vi "MotorTestBench_Main.vi"() -> ()   [LabVIEW 2026]
uses:
  MotorMeasurements.ctl
  FaultInjectionMode.ctl
  <vilib>/Plasmionique/MB Master/MB_Master_TCP/MB_Master_TCP.lvclass
  C:/Program Files/National Instruments/LabVIEW 2026/vi.lib/Plasmionique/MB Master/MB_Master/MB_Master.lvclass
panel:
  in  "Fault Injection":T1
  out "Modbus System Status":u16
  in  "Timeout":i32=10000
  in  "Slave ID":u8=255
  in  "Port":u16=502
  in  "IP Address":string="localhost"
  in  "Test Vibration \nLimit (mm/s)":dbl
  in  "Safety Vibration\nTrip (mm/s)":dbl
  out "Vibration OK":bool
  in  "Measurement\nSource":T2(ring)
  out "Measurements":T3
  in  "ai0 = Temperature\nai1 = Current\nai2 = Torque\nai3 = Vibration\nai4 = RPM":tag
  out "RPM Error":dbl
  out "Test Result":string
  in  "RESET TEST":bool
  in  "Safety Current\nTrip (A)":dbl
  in  "Safety Temp.\nTrip (°C)":dbl
  out "TEST FAILED":bool
  out "Current OK":bool
  out "RPM OK":bool
  in  "Test Current\nLimit (A)":dbl
  in  "RPM Tolerance":dbl
  out "Temprature OK":bool
  in  "Test Temperature\nLimit (°C)":dbl
  in  "START TEST":bool
  out "Current Test State":T4(ring)
  in  "STOP SYSTEM":bool
  # "SETTINGS"
  # "MOTOR TEST BENCH"
  # "DAQ Channel Selection"
  # "TEST CONTROL"
  # "LIVE MEASUREMENTS"
  # "LIMITS"
  # "MODBUS SETTINGS"
  # "FAULT / STATUS"
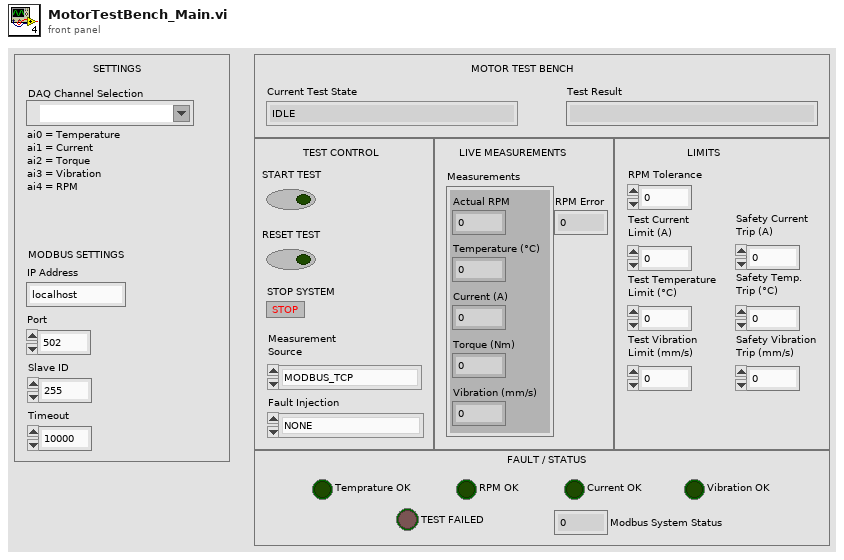
[diagram p1: front panel]
types:
  T1 = typedef "FaultInjectionMode.ctl" = enum16{"NONE", "OVERCURRENT", "OVERTEMPERATURE", "HIGH_VIBRATION", "RPM_SENSOR_FAILURE"}
  T2 = enum16{"MODBUS_TCP", "NI_DAQ", "SOFTWARE_SIMULATOR"}
  T3 = typedef "MotorMeasurements.ctl" = cluster{"Temperature (°C)":dbl, "Current (A)":dbl, "Torque (Nm)":dbl, "Vibration (mm/s)":dbl, "Actual RPM":dbl}
  T4 = enum16{"IDLE", "TEST_1000_RPM", "TEST_2000_RPM", "TEST_3000_RPM", "COMPLETE", "FAULT", "SHUTDOWN"}
  T5 = enum16{"open", "open or create", "create or replace", "create", "open (read-only)"}
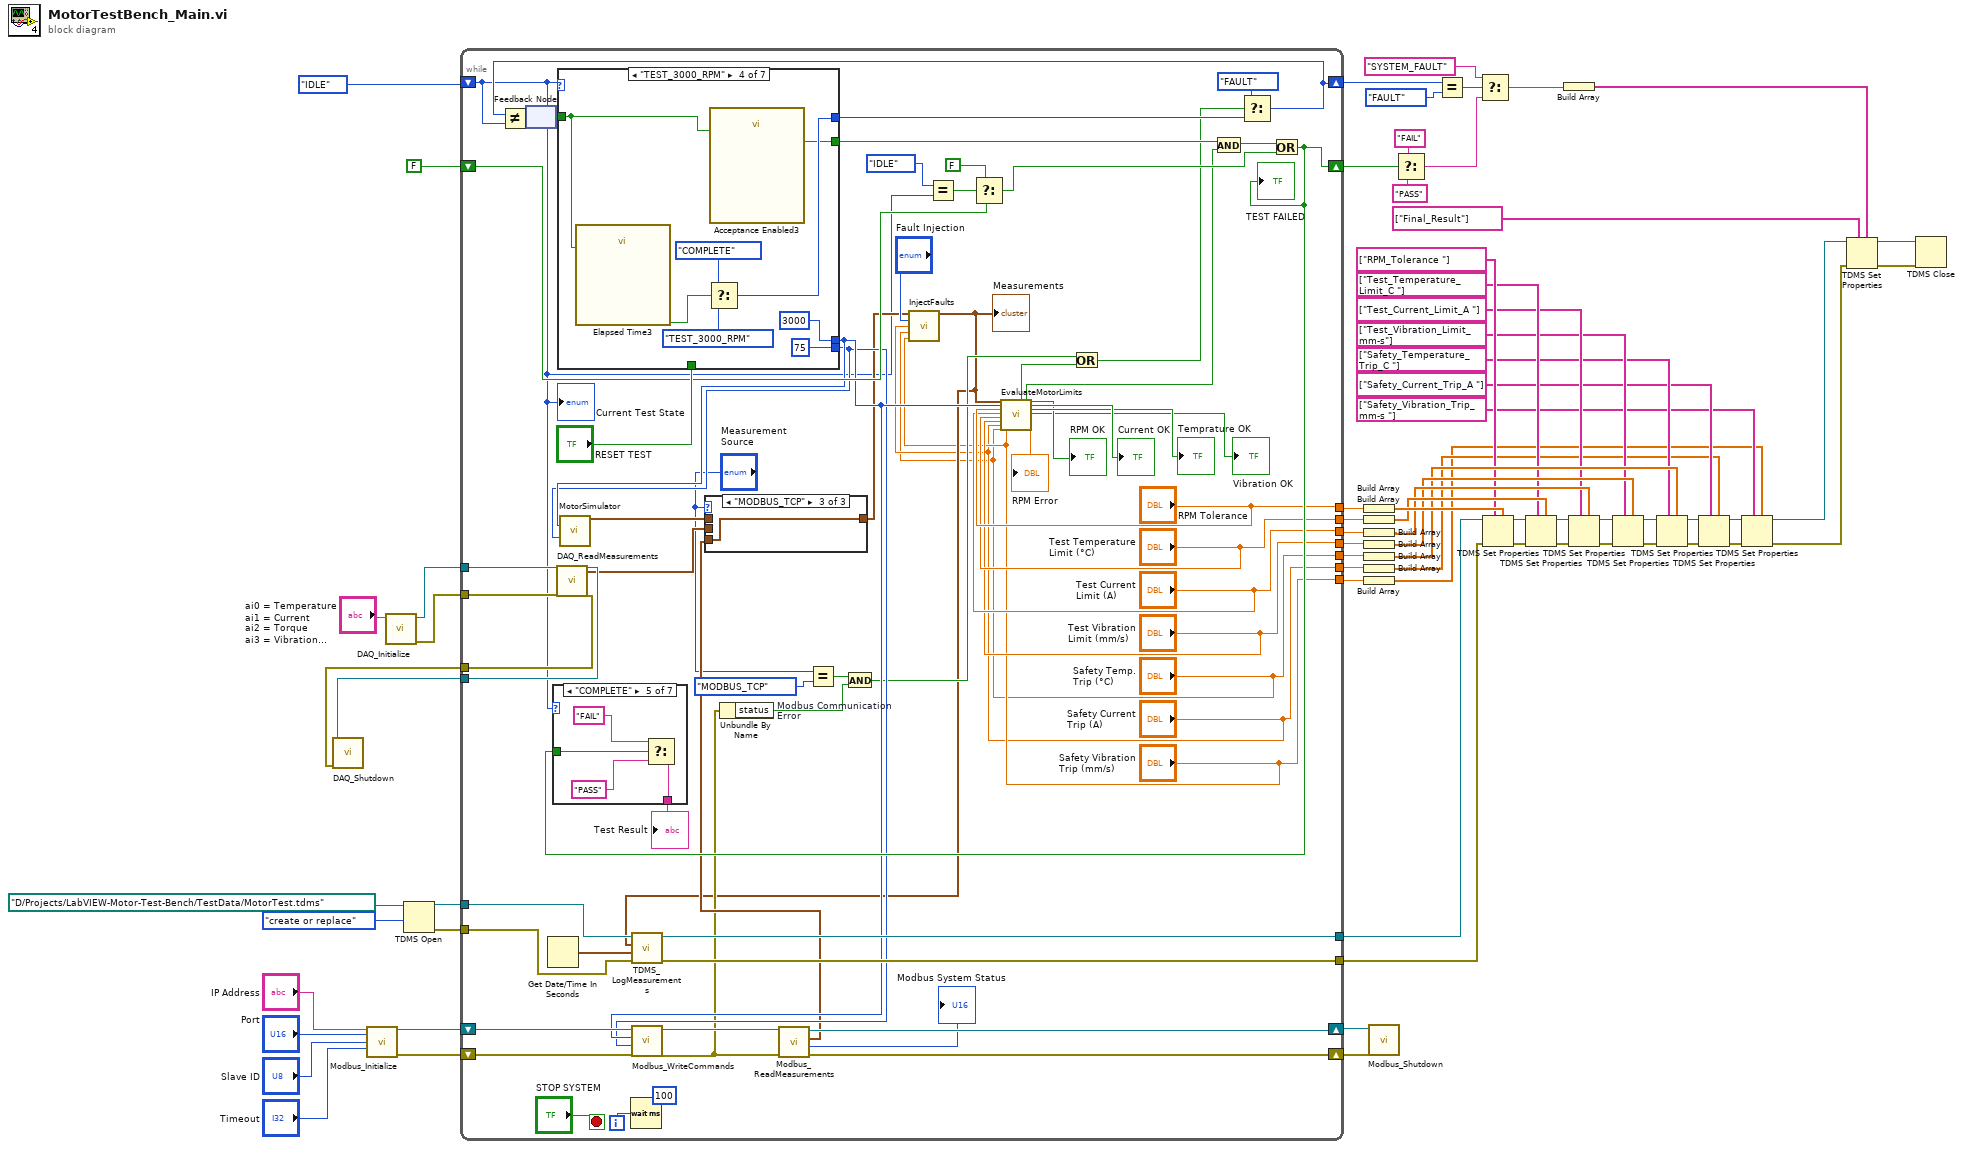
[diagram p0: block diagram]
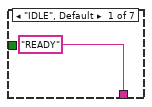
[diagram p4: hidden frame]
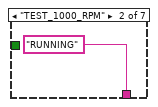
[diagram p5: hidden frame]
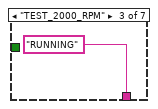
[diagram p6: hidden frame]
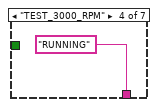
[diagram p7: hidden frame]
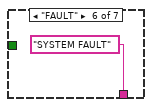
[diagram p8: hidden frame]
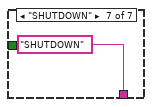
[diagram p9: hidden frame]
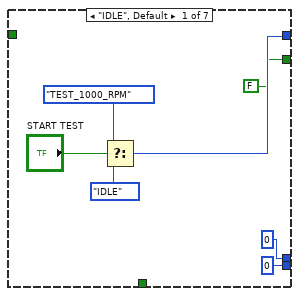
[diagram p10: hidden frame]
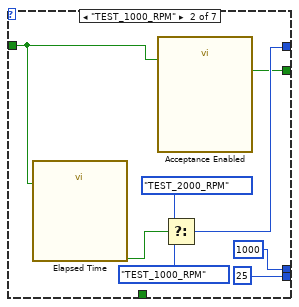
[diagram p11: hidden frame]
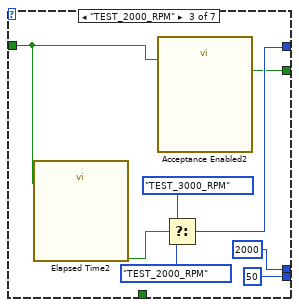
[diagram p12: hidden frame]
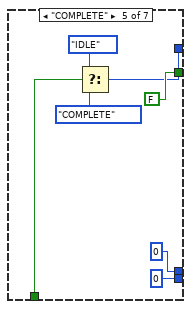
[diagram p13: hidden frame]
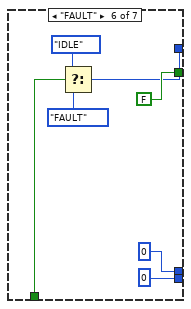
[diagram p14: hidden frame]
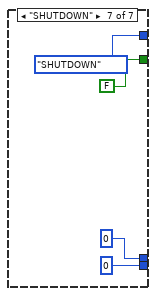
[diagram p15: hidden frame]
diagram:
  n1 = call "Modbus_Initialize.vi"("IP Address"="IP Address", "Port (502)"="Port", "Slave ID (255)"="Slave ID", "Timeout (10000)"="Timeout") -> ("MB_TCP session"=w6:refnum<class "MB_Master_TCP.lvclass">, "error out"=w4:errorcluster)  [unwired: 10 in]
  n2 = call "DAQ_Initialize.vi"("ai0 = Temperature\nai1 = Current\nai2 = Torque\nai3 = Vibration\nai4 = RPM"="ai0 = Temperature\nai1 = Current\nai2 = Torque\nai3 = Vibration\nai4 = RPM") -> ("error out"=w29:errorcluster, "task out"=w30:refnum<k21>)  [unwired: 9 in]
  n3 = TDMS Open(10:T5."create or replace" ("operation (0:open)"), 11:path "D:/Projects/LabVIEW-Motor-Test-Bench/TestData/MotorTest.tdms" ("file path")) -> (0:w66:errorcluster, 3:w67:refnum<k34>)  [unwired: 5 in]
  n4 = while {
    shift-right: [w73] -> w2
    shift-left: T4."IDLE" ("Enum") -> [w72]
    tunnel: w67 -> [w100]
    tunnel: [w98] -> w43
    tunnel: w66 -> [w99]
    tunnel: [w97] -> w42
    shift-right: [w122] -> w64
    shift-left: FALSE -> [w123]
    tunnel: ["RPM Tolerance"] -> w59
    tunnel: ["Test Temperature\nLimit (°C)"] -> w60
    tunnel: ["Test Current\nLimit (A)"] -> w61
    tunnel: ["Safety Temp.\nTrip (°C)"] -> w17
    tunnel: ["Safety Current\nTrip (A)"] -> w16
    tunnel: w30 -> [w113]
    tunnel: w29 -> [w112]
    tunnel: [w111] -> w28
    tunnel: [w110] -> w27
    tunnel: ["Test Vibration \nLimit (mm/s)"] -> w18
    tunnel: ["Safety Vibration\nTrip (mm/s)"] -> w15
    shift-right: [w90] -> w5
    shift-left: w6 -> [w96]
    shift-right: [w91] -> w3
    shift-left: w4 -> [w93]
    i -> [w130]
    stop <- "STOP SYSTEM" stop-if-true
    (unwired) u32 100 ("millisecond timer value")
    n5 = feedback #1() -> (w70:bool)  [unwired: 1 in]
    n6 = Get Date/Time In Seconds() -> (seconds since 1Jan1904=w101:timestamp)
    n7 = call "DAQ_ReadMeasurements.vi"("task/channels in"=w113, "error in"=w112) -> ("task out"=w111:refnum<k21>, "Measurements"=w109:T3, "error out"=w110:errorcluster)  [unwired: 18 in, 5 out]
    n8 = case shown="\"TEST_3000_RPM\"" w72 {
      tunnel: [w146 w154 w162 w171 w177 w184 T4."SHUTDOWN" ("Enum")] -> w114
      tunnel: [0 1000 2000 3000 0 0 0] -> w95
      tunnel: [0 25 50 75 0 0 0] -> w94
      tunnel: [FALSE w153 w161 w169 FALSE FALSE FALSE] -> w128
      tunnel: "RESET TEST" -> [_ _ _ _ w176 w183 _]
      tunnel: w70 -> [_ w152 w160 w168 _ _ _]
      frame "IDLE", Default {
        n9 = Select(t=T4."TEST_1000_RPM" ("Enum"), s="START TEST", f=T4."IDLE" ("Enum")) -> (s? t:f=w146:T4)
      }
      frame "TEST_1000_RPM" {
        n10 = call "Elapsed Time"("Reset"=w152) -> ("Time has Elapsed"=w157:bool)  [unwired: 11 in, 7 out]
        n11 = call "Acceptance Enabled"("Reset"=w152) -> ("Time has Elapsed"=w153:bool)  [unwired: 11 in, 7 out]
        n12 = Select(t=T4."TEST_2000_RPM" ("Enum"), s=w157, f=T4."TEST_1000_RPM" ("Enum")) -> (s? t:f=w154:T4)
      }
      frame "TEST_2000_RPM" {
        n13 = call "Elapsed Time2"("Reset"=w160) -> ("Time has Elapsed"=w165:bool)  [unwired: 11 in, 7 out]
        n14 = call "Acceptance Enabled2"("Reset"=w160) -> ("Time has Elapsed"=w161:bool)  [unwired: 11 in, 7 out]
        n15 = Select(t=T4."TEST_3000_RPM" ("Enum"), s=w165, f=T4."TEST_2000_RPM" ("Enum")) -> (s? t:f=w162:T4)
      }
      frame "TEST_3000_RPM" {
        n16 = call "Elapsed Time3"("Reset"=w168) -> ("Time has Elapsed"=w174:bool)  [unwired: 11 in, 7 out]
        n17 = Select(t=T4."COMPLETE" ("Enum"), s=w174, f=T4."TEST_3000_RPM" ("Enum")) -> (s? t:f=w171:T4)
        n18 = call "Acceptance Enabled3"("Reset"=w168) -> ("Time has Elapsed"=w169:bool)  [unwired: 11 in, 7 out]
      }
      frame "COMPLETE" {
        n19 = Select(t=T4."IDLE" ("Enum"), s=w176, f=T4."COMPLETE" ("Enum")) -> (s? t:f=w177:T4)
      }
      frame "FAULT" {
        n20 = Select(t=T4."IDLE" ("Enum"), s=w183, f=T4."FAULT" ("Enum")) -> (s? t:f=w184:T4)
      }
      frame "SHUTDOWN" {
      }
    }
    n21 = call "MotorSimulator.vi"("Commanded RPM"=w95, "Load (%)"=w94) -> ("Measurements"=w108:T3)  [unwired: 13 in]
    n22 = Wait (ms)(milliseconds to wait=w130) -> ()  [unwired: 1 out]
    n23 = call "Modbus_WriteCommands.vi"("error in (no error)"=w93, "Load (%)"=w94, "Commanded RPM"=w95, "MB session in"=w96) -> ("error out"=w84:errorcluster, "MB session out"=w92:refnum<class "MB_Master_TCP.lvclass">)  [unwired: 6 in]
    n24 = Unbundle By Name "Modbus Communication \nError"(w84) -> ("status"=w83:bool)
    n25 = call "Modbus_ReadMeasurements.vi"("error in (no error)"=w84, "MB session in"=w92) -> ("error out"=w91:errorcluster, "System \nStatus"=→"Modbus System Status":u16, "Measurements"=w88:T3, "MB session out"=w90:refnum<class "MB_Master_TCP.lvclass">)  [unwired: 6 in]
    n26 = case shown="\"MODBUS_TCP\"" "Measurement\nSource" {
      tunnel: w109 -> [w132 _ _]
      tunnel: w108 -> [_ w133 _]
      tunnel: [w132 w133 w134] -> w79
      tunnel: w88 -> [_ _ w134]
      frame "NI_DAQ", Default {
      }
      frame "SOFTWARE_SIMULATOR" {
      }
      frame "MODBUS_TCP" {
      }
    }
    n27 = Equal?(x="Measurement\nSource", y=T2."MODBUS_TCP" ("Measurement\nSource 2")) -> (x = y?=w85:bool)
    n28 = And(x=w85, y=w83) -> (x .and. y?=w81:bool)
    n29 = call "InjectFaults.vi"("MotorMeasurements"=w79, "Fault Injection"="Fault Injection", "Safety Current Trip"="Safety Current\nTrip (A)", "Safety Temperature Trip"="Safety Temp.\nTrip (°C)", "Safety Vibration Trip"="Safety Vibration\nTrip (mm/s)") -> ("Modified Measurements"=w78:T3)  [unwired: 9 in, 1 out]
    "Measurements" <- w78
    n30 = call "TDMS_LogMeasurements.vi"("error in (no error)"=w99, "Current Time"=w101, "Motor Measurements"=w78, "tdms file"=w100) -> ("error out"=w97:errorcluster, "tdms file out"=w98:refnum<k34>)  [unwired: 6 in]
    n31 = Equal?(x=T4."IDLE" ("Enum"), y=w72) -> (x = y?=w125:bool)
    n32 = Select(t=FALSE, s=w125, f=w123) -> (s? t:f=w116:bool)
    n33 = call "EvaluateMotorLimits.vi"("MotorMeasurements"=w78, "Commanded RPM"=w95, "RPM Tolerance"="RPM Tolerance", "Test Current Limit (A)"="Test Current\nLimit (A)", "Test Temperature Limit (°C)"="Test Temperature\nLimit (°C)", "Test Vibration Limit (mm/s)"="Test Vibration \nLimit (mm/s)", "Safety Current Trip (A)"="Safety Current\nTrip (A)", "Safety Temperature Trip (°C)"="Safety Temp.\nTrip (°C)", "Safety Vibration Trip (mm/s)"="Safety Vibration\nTrip (mm/s)") -> ("SYSTEM FAULT REQUEST"=w82:bool, "CURRENT SAMPLE FAILED"=w106:bool, "RPM OK"=→"RPM OK":bool, "CURRENT OK"=→"Current OK":bool, "TEMPERATURE OK"=→"Temprature OK":bool, "VIBRATION OK"=→"Vibration OK":bool, "RPM Error"=→"RPM Error":dbl)  [unwired: 9 in, 3 out]
    n34 = Or(x=w81, y=w82) -> (x .or. y?=w77:bool)
    n35 = And(x=w128, y=w106) -> (x .and. y?=w117:bool)
    n36 = Select(t=T4."FAULT" ("Enum"), s=w77, f=w114) -> (s? t:f=w73:T4)
    n37 = Not Equal?(x=w73, y=w72) -> (x != y?=w71:bool)
    n38 = feedback-in #1(w71) -> ()
    n39 = Or(x=w117, y=w116) -> (x .or. y?=w122:bool)
    "TEST FAILED" <- w122
    n40 = case shown="\"COMPLETE\"" w72 {
      tunnel: ["READY" "RUNNING" "RUNNING" "RUNNING" w139 "SYSTEM FAULT" "SHUTDOWN"] -> w121
      tunnel: w122 -> [_ _ _ _ w140 _ _]
      frame "IDLE", Default {
      }
      frame "TEST_1000_RPM" {
      }
      frame "TEST_2000_RPM" {
      }
      frame "TEST_3000_RPM" {
      }
      frame "COMPLETE" {
        n41 = Select(t="FAIL", s=w140, f="PASS") -> (s? t:f=w139:string)
      }
      frame "FAULT" {
      }
      frame "SHUTDOWN" {
      }
    }
    "Test Result" <- w121
    "Current Test State" <- w72
  }
  n42 = call "DAQ_Shutdown.vi"("error in"=w27, "task/channels in"=w28) -> ()  [unwired: 9 in, 1 out]
  n43 = Build Array(w59) -> (w58:dbl[])
  n44 = Build Array(w60) -> (w57:dbl[])
  n45 = Build Array(w61) -> (w56:dbl[])
  n46 = Build Array(w18) -> (w55:dbl[])
  n47 = Build Array(w17) -> (w54:dbl[])
  n48 = Build Array(w16) -> (w14:dbl[])
  n49 = Build Array(w15) -> (w13:dbl[])
  n50 = call "Modbus_Shutdown.vi"("MB session in"=w5, "error in (no error)"=w3) -> ()  [unwired: 8 in, 1 out]
  n51 = Select(t="FAIL", s=w64, f="PASS") -> (s? t:f=w34:string)
  n52 = Equal?(x=w2, y=T4."FAULT" ("Enum")) -> (x = y?=w36:bool)
  n53 = Select(t="SYSTEM_FAULT", s=w36, f=w34) -> (s? t:f=w33:string)
  n54 = TDMS Set Properties(5:w58, 7:string[] ["RPM_Tolerance "] ("property names"), 8:w42, 11:w43) -> (0:w41:errorcluster, 3:w47:refnum<k34>)  [unwired: 2 in, 2 out]
  n55 = TDMS Set Properties(5:w57, 7:string[] ["Test_Temperature_Limit_C "] ("property names"), 8:w41, 11:w47) -> (0:w40:errorcluster, 3:w46:refnum<k34>)  [unwired: 2 in, 2 out]
  n56 = Build Array(w33) -> (w35:string[])
  n57 = TDMS Set Properties(5:w56, 7:string[] ["Test_Current_Limit_A "] ("property names"), 8:w40, 11:w46) -> (0:w39:errorcluster, 3:w45:refnum<k34>)  [unwired: 2 in, 2 out]
  n58 = TDMS Set Properties(5:w55, 7:string[] ["Test_Vibration_Limit_mm-s"] ("property names"), 8:w39, 11:w45) -> (0:w38:errorcluster, 3:w44:refnum<k34>)  [unwired: 2 in, 2 out]
  n59 = TDMS Set Properties(5:w54, 7:string[] ["Safety_Temperature_Trip_C "] ("property names"), 8:w38, 11:w44) -> (0:w25:errorcluster, 3:w26:refnum<k34>)  [unwired: 2 in, 2 out]
  n60 = TDMS Set Properties(5:w14, 7:string[] ["Safety_Current_Trip_A "] ("property names"), 8:w25, 11:w26) -> (0:w23:errorcluster, 3:w24:refnum<k34>)  [unwired: 2 in, 2 out]
  n61 = TDMS Set Properties(5:w13, 7:string[] ["Safety_Vibration_Trip_mm-s "] ("property names"), 8:w23, 11:w24) -> (0:w11:errorcluster, 3:w12:refnum<k34>)  [unwired: 2 in, 2 out]
  n62 = TDMS Set Properties(5:w35, 7:string[] ["Final_Result"] ("property names"), 8:w11, 11:w12) -> (0:w48:errorcluster, 3:w49:refnum<k34>)  [unwired: 2 in, 2 out]
  n63 = TDMS Close(8:w48, 11:w49) -> ()  [unwired: 2 out]
